vi "GetSavedTCP.vi"(8 "error in":errorcluster, 10 "Channels to Acq":i32=1, 11 "ActiveDSO In":refnum<k7>) -> (0 "error out":errorcluster, 1 "Samp Rate":sgl format="%.2e", 3 "Active DSO out":refnum<k7>, 5 "Att (dB)":dbl[](array[numeric]) format="%.2f")   [LabVIEW 2022 SP3]
uses:
  Motion Controllers/-MotionRoutines/MotionGlobals.vi
panel:
  in  "address":string="IP:65.246.218.103"
  out "FS Volt pp":dbl format="%.2f"
  out "V/ div":string
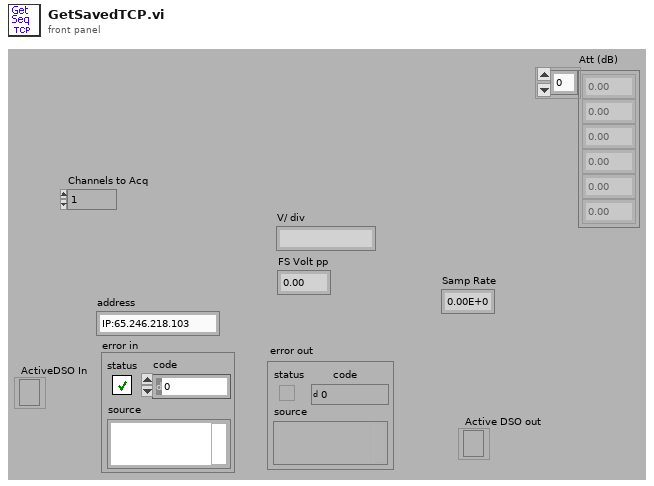
[diagram p1: front panel]
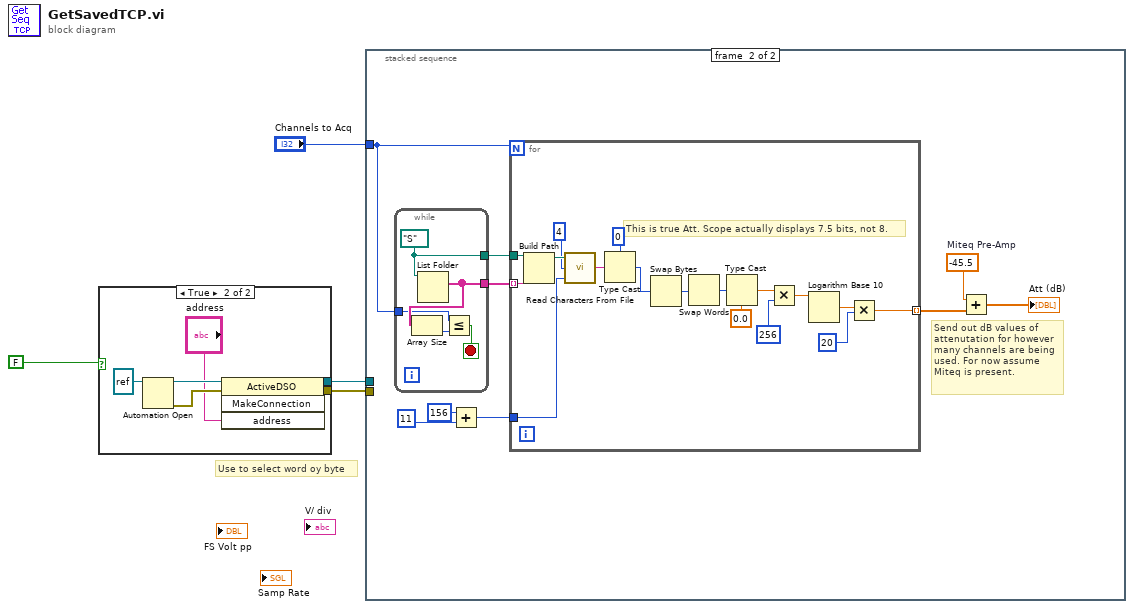
[diagram p0: block diagram]
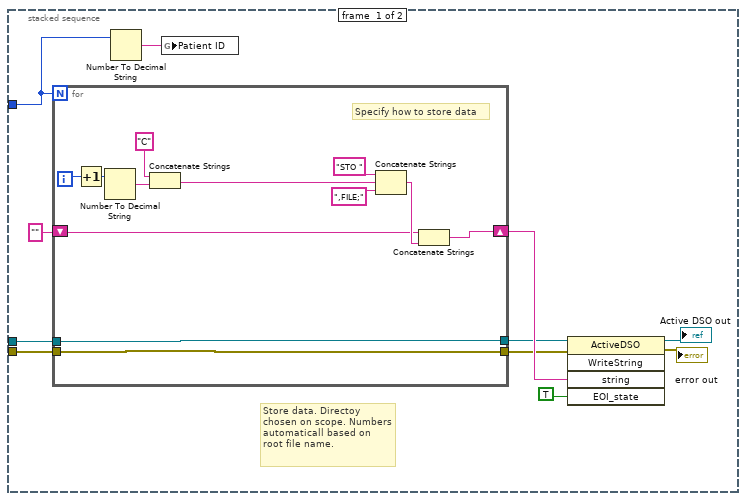
[diagram p2: hidden frame]
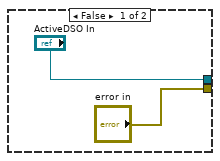
[diagram p3: hidden frame]
diagram:
  # "Use to select word oy byte"
  n1 = case shown="True" FALSE ("Case Constant\n(See Context Help)") {
    tunnel: ["ActiveDSO In" w8] -> w2
    tunnel: ["error in" w9] -> w1
    frame False {
    }
    frame True {
      n2 = Automation Open(Automation Refnum=refnum<k7> refnum ("ACTIVEDSOLib.ActiveDSO")) -> (Automation Refnum=w11:refnum<k7>, error out=w12:errorcluster)  [unwired: 1 in, 2 out]
      n3 = invoke class="ActiveDSO" method="MakeConnection"(reference=w11, error in=w12, "address"="address") -> (reference out=w8:refnum<k7>, error out=w9:errorcluster)  [unwired: 1 in, 2 out]
    }
  }
  n4 = stacked-sequence {
    tunnel: w2 -> [w22 _]
    tunnel: w1 -> [w21 _]
    tunnel: "Channels to Acq" -> [w20 w39]
    frame #0 {
      # "Store data. Directoy chosen on scope. Numbers automaticall based on root file name."
      n5 = for {
        N: w20 -> [_]
        tunnel: w22 -> [w25]
        tunnel: w21 -> [w24]
        shift-right: [w26] -> w15
        shift-left: "" -> [w27]
        tunnel: [w25] -> w14
        tunnel: [w24] -> w13
        i -> [w31]
        # "Specify how to store data"
        n6 = Increment(x=w31) -> (x+1=w32:i32)
        n7 = Number To Decimal String(number=w32) -> (decimal integer string=w33:string)  [unwired: 1 out]
        n8 = Concatenate Strings("C", w33) -> (w34:string)
        n9 = Concatenate Strings("STO ", w34, ",FILE;") -> (w28:string)
        n10 = Concatenate Strings(w27, w28) -> (w26:string)
      }
      n11 = Number To Decimal String(number=w20) -> (decimal integer string=w23:string)  [unwired: 1 out]
      n12 = global write "MotionGlobals.vi" "Patient ID"(w23) -> ()
      n13 = invoke class="ActiveDSO" method="WriteString"(reference=w14, error in=w13, "string"=w15, "EOI_state"=TRUE) -> (reference out=→"Active DSO out":refnum<k7>, error out=→"error out":errorcluster)  [unwired: 1 in, 3 out]
    }
    frame #1 {
      w41 = -45.5  # Miteq Pre-Amp
      # "Send out dB values of attenutation for however many channels are being used. For now assume Miteq is present."
      n14 = while {
        tunnel: [w65] -> w43
        tunnel: [w66] -> w42
        tunnel: w39 -> [w62]
        stop <- w63 stop-if-true
        w66 = path "S:/" ("file path (dialog if empty)")
        n15 = List Folder(path=w66) -> (filenames=w65:string[])  [unwired: 1 in, 5 out]
        n16 = Array Size(array=w65) -> (size(s)=w64:i32)
        n17 = Less Or Equal?(x=w62, y=w64) -> (x <= y?=w63:bool)
      }
      n18 = Add(x=156, y=11 ("Offset")) -> (x+y=w36:i32)
      n19 = for {
        N: w39 -> [_]
        tunnel: w42 -> [w61]
        tunnel: w43 -> [w60] mode=indexing
        tunnel: [w55] -> w44 mode=indexing
        tunnel: w36 -> [w53]
        # "This is true Att. Scope actually displays 7.5 bits, not 8."
        n20 = Build Path(base path=w61, name or relative path=w60) -> (appended path=w54:path)
        n21 = call <vilib>:"Read Characters From File.vi"("file path (dialog if empty)"=w54, "number of characters (all:-1)"=4, "start of read offset (chars.:0)"=w53) -> ("character string"=w47:string)  [unwired: 6 out]
        n22 = Type Cast(type=0, x=w47) -> (*(type *) &x=w50:i32)
        n23 = Swap Bytes(anything=w50) -> (byte swapped=w48:i32)
        n24 = Swap Words(1:w48) -> (0:w51:i32)
        n25 = Type Cast(type=sgl 0.0, x=w51) -> (*(type *) &x=w45:sgl)
        n26 = Multiply(x=w45, y=256) -> (x*y=w59:sgl)
        n27 = Logarithm Base 10(1:w59) -> (0:w57:sgl)
        n28 = Multiply(x=w57, y=20) -> (x*y=w55:sgl)
      }
      n29 = Add(x=w41, y=w44) -> (x+y=→"Att (dB)":dbl[])
    }
  }
